vi "FeedBack Chanel.vi"(0 "Test Name":string, 5 "Channels (Int)":i32[](array[numeric]), 7 "FeedBack Channel":string[](array[string])=["fgdgfvcbc", "vnfhgjkn", "21354682"], 9 "Wait/Poll (ms)":u32, 11 "Parameter":u8) -> (4 "Out":i32, 6 "Array":bool[](array[boolean]), 12 "Input Status":bool[](array[boolean]), 13 "Channel No":i32[](array[numeric]))   [LabVIEW 2015]
uses:
  Galobal variable_TI.vi
panel:
  out "Pokayoka Result":cluster{"Sensor Name":string, "Boolean":bool}[](array[cluster])
  out "output array":bool[](array[boolean])
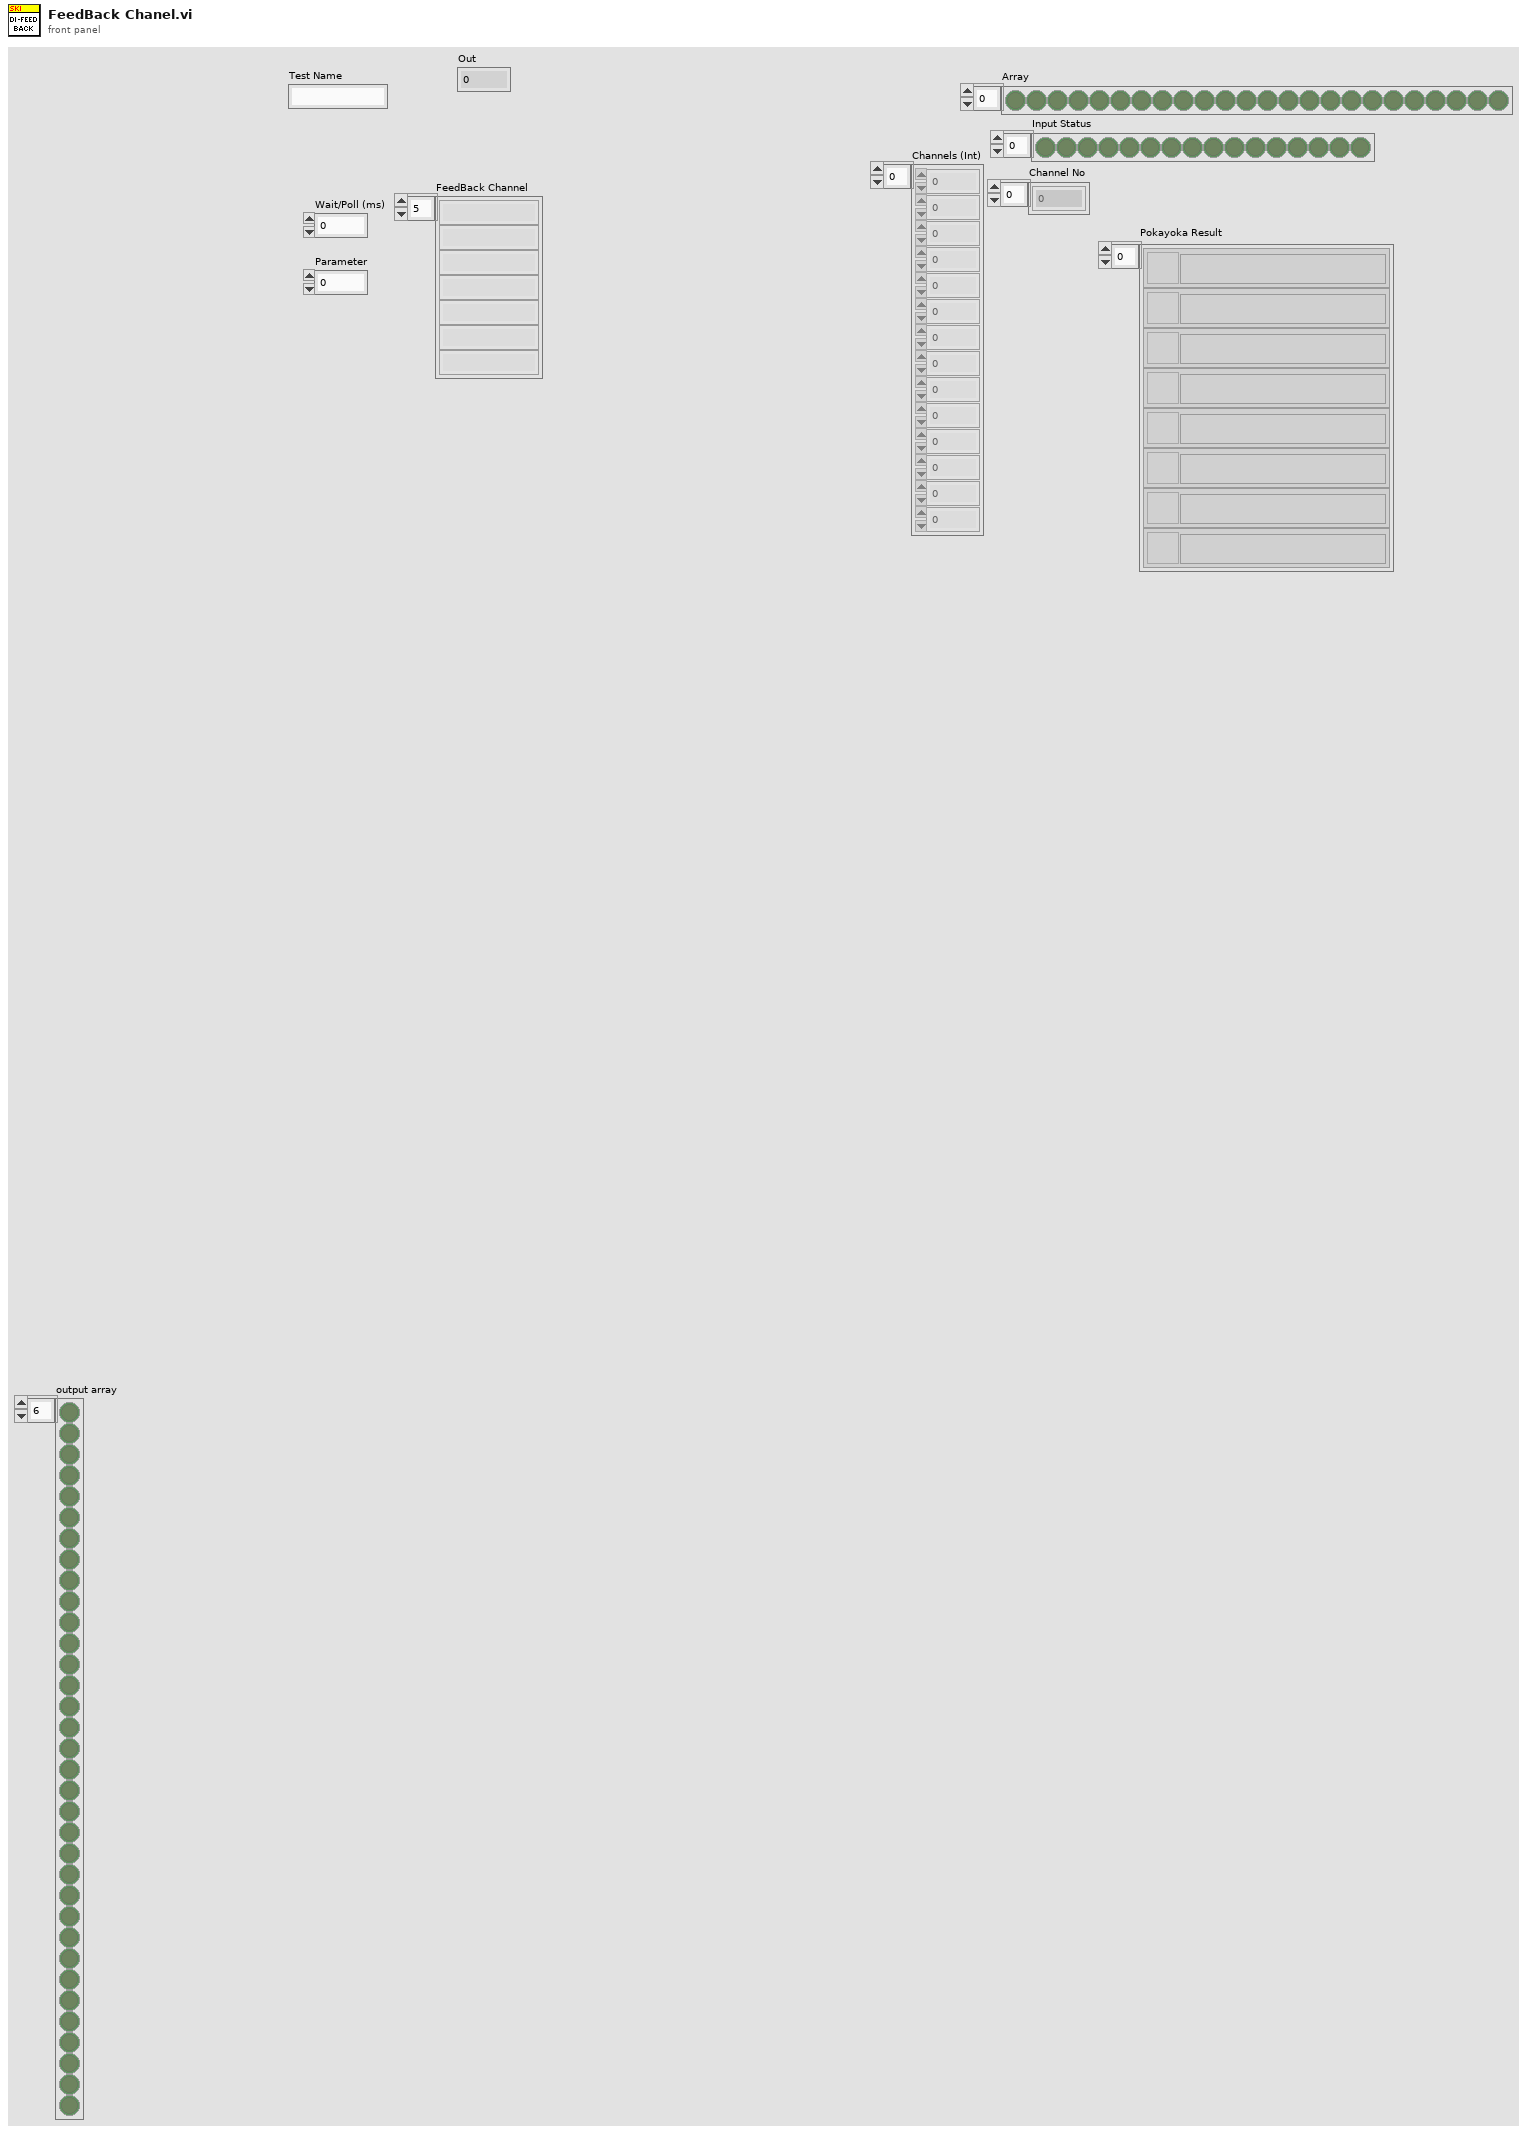
[diagram p1: front panel]
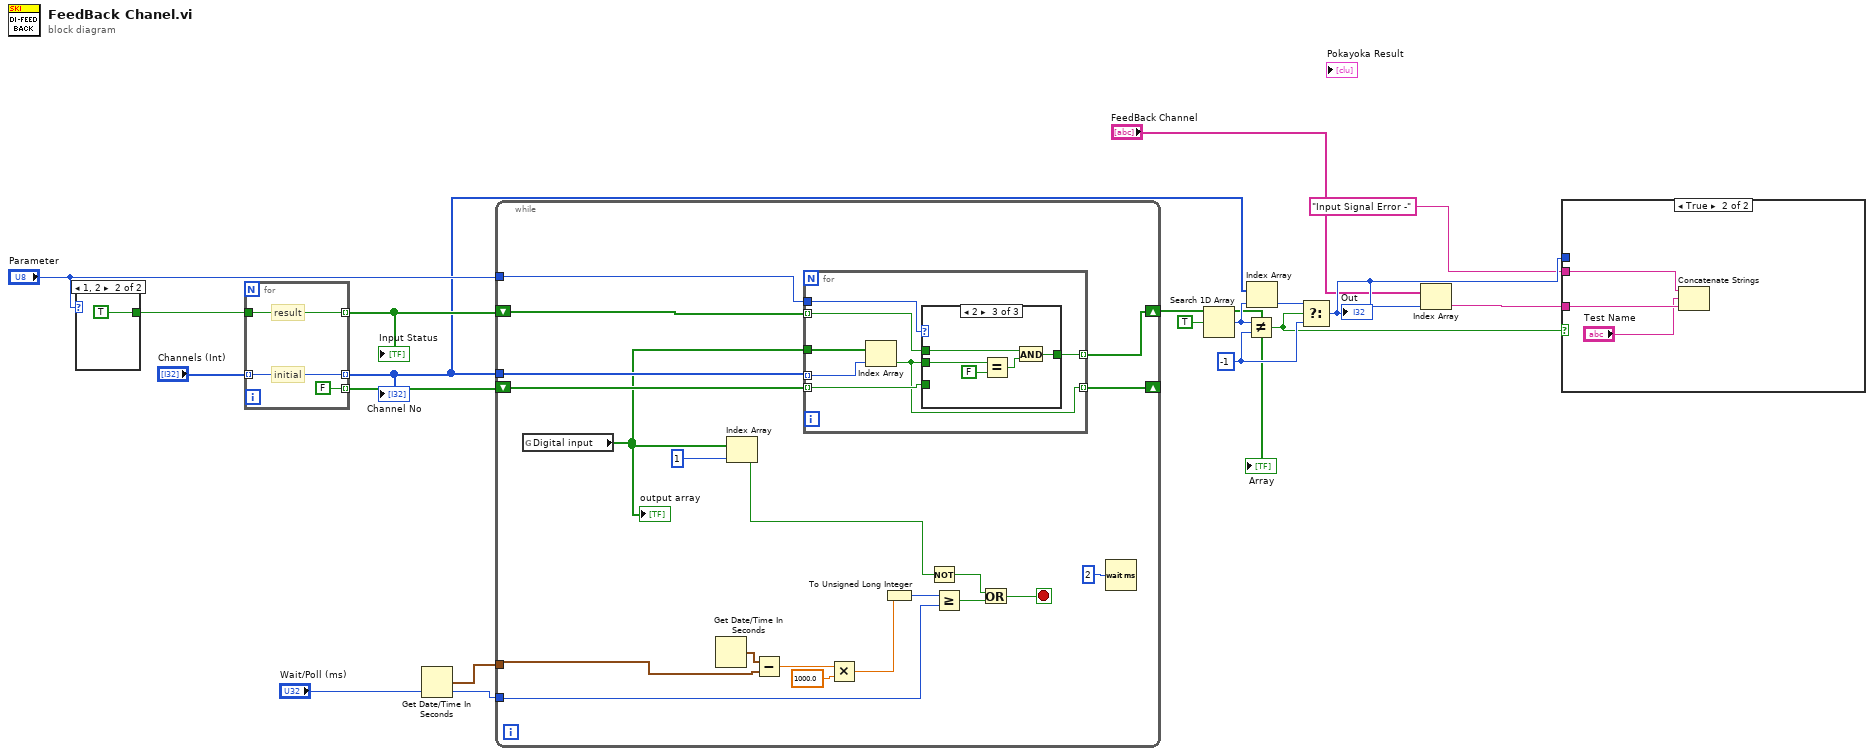
[diagram p0: block diagram]
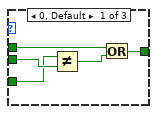
[diagram p3: hidden frame]
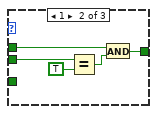
[diagram p4: hidden frame]
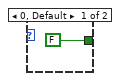
[diagram p5: hidden frame]
diagram:
  w18 = -1 ("y")
  n1 = case shown="1, 2" "Parameter" {
    tunnel: [FALSE TRUE] -> w8
    frame 0, Default {
    }
    frame 1, 2 {
    }
  }
  n2 = for {
    tunnel: [w23] -> w3 mode=indexing
    tunnel: w8 -> [w23]
    tunnel: "Channels (Int)" -> [w22] mode=indexing
    tunnel: [w22] -> w2 mode=indexing
    tunnel: [FALSE] -> w13 mode=indexing
    # "result"
    # "initial"
  }
  "Input Status" <- w3
  "Channel No" <- w2
  n3 = Get Date/Time In Seconds() -> (seconds since 1Jan1904=w11:timestamp)
  n4 = while {
    tunnel: "Wait/Poll (ms)" -> [w28]
    tunnel: w11 -> [w42]
    tunnel: w2 -> [w37]
    tunnel: "Parameter" -> [w36]
    shift-right: [w35] -> w15
    shift-left: w3 -> [w33]
    shift-right: [w34] -> _
    shift-left: w13 -> [w32]
    stop <- w30 stop-if-true
    n5 = global read "Galobal variable_TI.vi" "Digital input"() -> (w24:bool[])
    "output array" <- w24
    n6 = Get Date/Time In Seconds() -> (seconds since 1Jan1904=w43:timestamp)
    n7 = Index Array(array=w24, index=1) -> (element=w26:bool)
    n8 = Subtract(x=w43, y=w42) -> (x-y=w41:dbl)
    n9 = for {
      tunnel: w32 -> [w45] mode=indexing
      tunnel: w33 -> [w47] mode=indexing
      tunnel: w24 -> [w50]
      tunnel: w37 -> [w49] mode=indexing
      tunnel: w36 -> [w48]
      tunnel: [w46] -> w35 mode=indexing
      tunnel: [w44] -> w34 mode=indexing
      n10 = Index Array(array=w50, index=w49) -> (element=w44:bool)
      n11 = case shown="2" w48 {
        tunnel: w44 -> [w55 w58 w65]
        tunnel: w47 -> [w53 w57 w62]
        tunnel: [w51 w56 w61] -> w46
        tunnel: w45 -> [w54 _ _]
        frame 0, Default {
          n12 = Not Equal?(x=w54, y=w55) -> (x != y?=w52:bool)
          n13 = Or(x=w53, y=w52) -> (x .or. y?=w51:bool)
        }
        frame 1 {
          n14 = Equal?(x=w58, y=TRUE) -> (x = y?=w59:bool)
          n15 = And(x=w57, y=w59) -> (x .and. y?=w56:bool)
        }
        frame 2 {
          n16 = Equal?(x=w65, y=FALSE) -> (x = y?=w63:bool)
          n17 = And(x=w62, y=w63) -> (x .and. y?=w61:bool)
        }
      }
    }
    n18 = Multiply(x=w41, y=1000.0) -> (x*y=w39:dbl)
    n19 = To Unsigned Long Integer(number=w39) -> (unsigned 32bit integer=w38:u32)
    n20 = Not(x=w26) -> (.not. x?=w27:bool)
    n21 = Greater Or Equal?(x=w38, y=w28) -> (x >= y?=w31:bool)
    n22 = Or(x=w27, y=w31) -> (x .or. y?=w30:bool)
    n23 = Wait (ms)(milliseconds to wait=u32 2) -> ()  [unwired: 1 out]
  }
  "Array" <- w15
  n24 = Search 1D Array(1D array=w15, element=TRUE) -> (index of element=w16:i32)  [unwired: 1 in]
  n25 = Not Equal?(x=w16, y=w18) -> (x != y?=w7:bool)
  n26 = Index Array(array=w2, index=w16) -> (element=w17:i32)
  n27 = Select(t=w17, s=w7, f=w18) -> (s? t:f=w6:i32)
  "Out" <- w6
  n28 = Index Array(array="FeedBack Channel", index=w6) -> (element=w5:string)
  n29 = case shown="True" w7 {
    tunnel: w6 -> [_ _]
    tunnel: w5 -> [_ w68]
    tunnel: "Input Signal Error -" ("string") -> [_ w66]
    frame False {
    }
    frame True {
      n30 = Concatenate Strings(w66, "Test Name", w68) -> ()  [unwired: 1 out]
    }
  }
